vi "Configure Acquisition Type.vi"(7 "Number Of Averages (8)":i32=8, 8 "error in (no error)":errorcluster, 9 "Acquisition Mode (0: Real time)":i32(ring) items=["Real time ", "Equivalent time"], 10 "Acquisition Type (0: Normal)":i32(ring) items=["Normal", "Peak Detect", "Average", "High Resolution"], 11 "VISA resource name":refnum<visa-resource-name>) -> (0 "error out":errorcluster, 3 "VISA resource name out":refnum<visa-resource-name>)   [LabVIEW 2017, in "Agilent 6000 Series.lvlib"]
doc: "This VI configures how the oscilloscope acquires data and fills the waveform record."
uses:
  <instrlib>/Agilent 6000 Series/Agilent 6000 Series.lvlib
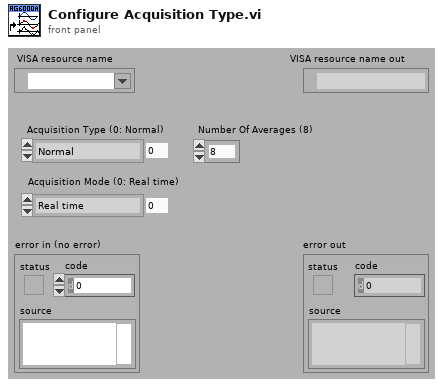
[diagram p1: front panel]
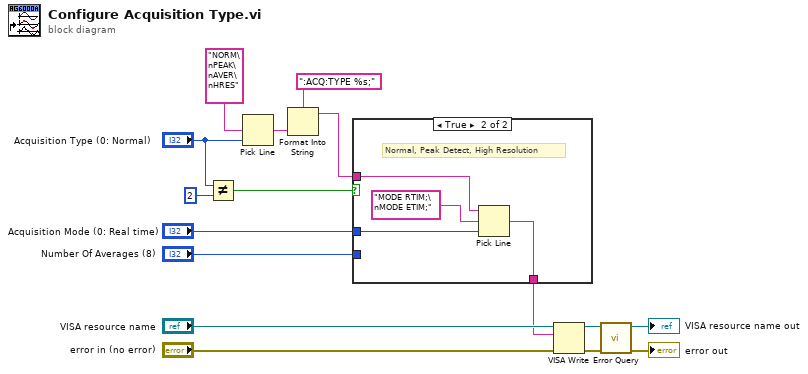
[diagram p0: block diagram]
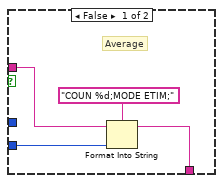
[diagram p2: hidden frame]
diagram:
  n1 = Not Equal?(x="Acquisition Type (0: Normal)", y=2) -> (x != y?=w2:bool)
  n2 = Pick Line(multi-line string="NORM\nPEAK\nAVER\nHRES", line index="Acquisition Type (0: Normal)") -> (output string=w8:string)  [unwired: 1 in]
  n3 = Format Into String(format string=":ACQ:TYPE %s;", w8) -> (resulting string=w4:string)  [unwired: 2 in, 1 out]
  n4 = case shown="True" w2 {
    tunnel: "Acquisition Mode (0: Real time)" -> [_ w24]
    tunnel: w4 -> [w19 w23]
    tunnel: [w18 w21] -> w3
    tunnel: "Number Of Averages (8)" -> [w20 _]
    frame False {
      # "Average"
      n5 = Format Into String(format string="COUN %d;MODE ETIM;", initial string=w19, w20) -> (resulting string=w18:string)  [unwired: 1 in, 1 out]
    }
    frame True {
      # "Normal, Peak Detect, High Resolution"
      n6 = Pick Line(string ("")=w23, multi-line string="MODE RTIM;\nMODE ETIM;", line index=w24) -> (output string=w21:string)
    }
  }
  n7 = VISA Write(VISA resource name="VISA resource name", write buffer=w3, error in (no error)="error in (no error)") -> (VISA resource name out=w12:refnum<visa-resource-name>, error out=w11:errorcluster)  [unwired: 1 out]
  n8 = call <instrlib>:"Error Query.vi"("error in (no error)"=w11, "VISA resource name"=w12) -> ("error out"=→"error out":errorcluster, "VISA resource name out"=→"VISA resource name out":refnum<visa-resource-name>)  [unwired: 6 in, 2 out]
